vi "Measure Channel.vi"(8 "error in":errorcluster, 10 "Selected Channel":T1, 11 "SimELoad in":refnum<class "SimEload.lvclass">) -> (0 "error out":errorcluster, 3 "SimELoad out":refnum<class "SimEload.lvclass">)   [LabVIEW 2019, in "SimELoad.lvlib" / "SimEload.lvclass"]
uses:
  SimEload.lvclass
  builds/Instruments/Electronic Load.lvlibp/Custom Controls/Channel Select.ctl
  C:/Users/Public/Documents/Development/builds/Instruments/Electronic Load.lvlibp/Electronic Load.lvclass
  builds/Instruments/Electronic Load.lvlibp/Accessors/Read Measurement Array.vi
  builds/Instruments/Electronic Load.lvlibp/Accessors/Write Measurement Array.vi
  builds/Instruments/Electronic Load.lvlibp/Electronic Load.lvclass
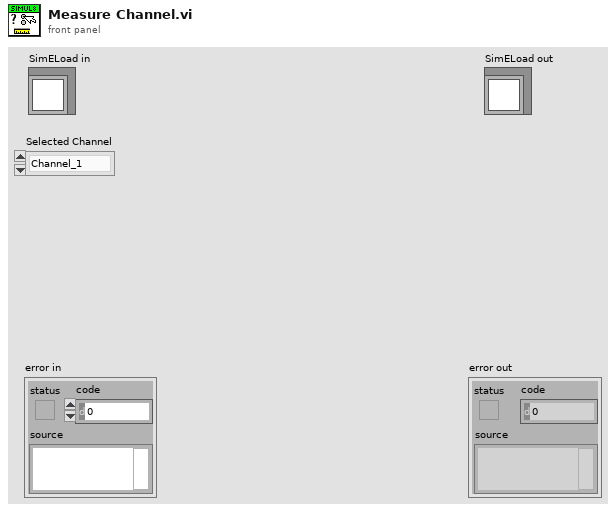
[diagram p1: front panel]
types:
  T1 = typedef "Electronic Load.lvlibp/Electronic Load.lvclass/Channel Select.ctl" = enum16{"Channel_1", "Channel_2", "Channel_3", "Channel_4", "Channel_5", "Channel_6"}
  T2 = typedef "Electronic Load.lvlibp/Electronic Load.lvclass/Measured Values.ctl" = cluster{"Output?":bool, "Current":dbl, "Voltage":dbl, "Power":dbl, "Channel Status":i32}
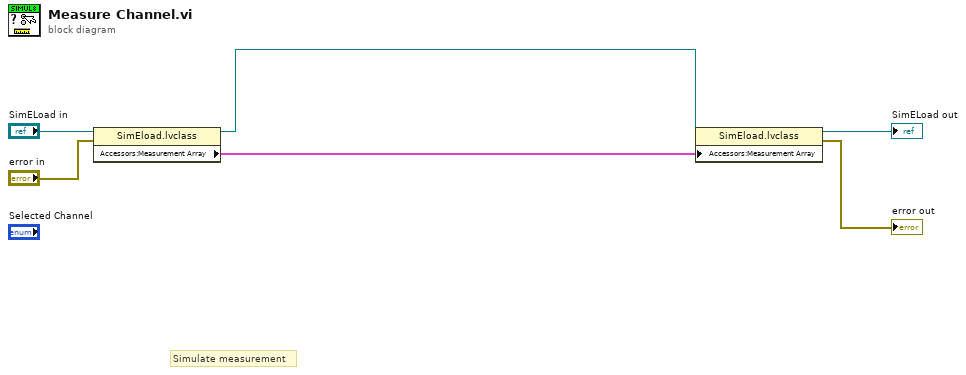
[diagram p0: block diagram]
diagram:
  # "Simulate measurement"
  n1 = property class="SimEload.lvclass"(reference="SimELoad in", error in="error in") -> (reference out=w5:refnum<class "SimEload.lvclass">, "Accessors:Measurement Array"=w1:T2[])  [unwired: 1 out]
  n2 = property class="SimEload.lvclass"(reference=w5, "Accessors:Measurement Array"=w1) -> (reference out=→"SimELoad out":refnum<class "SimEload.lvclass">, error out=→"error out":errorcluster)  [unwired: 1 in]
